vi "Read me and Help.vi"(7 "path":path, 11 "error in":errorcluster) -> (15 "error out":errorcluster)   [LabVIEW 2012]
uses:
  <vilib>/Platform/browser.llb/Open URL in Default Browser (path).vi
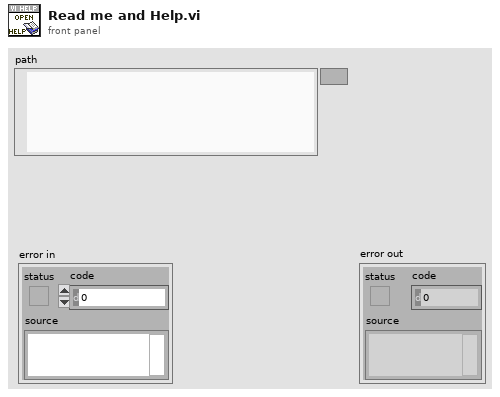
[diagram p1: front panel]
types:
  T1 = enum32{"Invalid", "Standard", "Closed", "Hidden", "Minimized", "Maximized"}
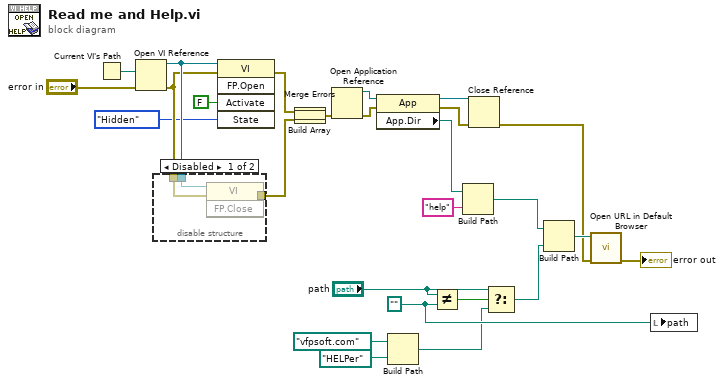
[diagram p0: block diagram]
diagram:
  w12 = path ""
  n1 = Current VI's Path() -> (path=w11:path)
  n2 = Open VI Reference(vi path=w11, error in (no error)="error in") -> (vi reference=w6:refnum<vi>, error out=w5:errorcluster)  [unwired: 4 in]
  n3 = disable-structure shown="Disabled" {
    disable-tunnel: w6 -> [w30 _]
    disable-tunnel: w5 -> [w29 w31]
    disable-tunnel: [w28 w31] -> w10
    frame Disabled {
      n4 = invoke class="VI" method="FP.Close"(reference=w30, error in=w29) -> (error out=w28:errorcluster)  [unwired: 1 in, 2 out]
    }
    frame Enabled {
    }
  }
  n5 = invoke class="VI" method="FP.Open"(reference=w6, error in=w5, "Activate"=FALSE ("Activate?"), "State"=T1."Hidden") -> (error out=w4:errorcluster)  [unwired: 1 in, 4 out]
  n6 = Build Array(w4, w10) -> (w7:errorcluster[])
  n7 = Merge Errors(w7) -> (w8:errorcluster)
  n8 = Open Application Reference(8:w8) -> (0:w21:errorcluster, 3:w20:refnum<vi>)  [unwired: 3 in]
  n9 = property class="App"(reference=w20, error in=w21) -> (reference out=w22:refnum<vi>, error out=w23:errorcluster, "App.Dir"=w24:path)
  n10 = Build Path(base path=path "vfpsoft.com" ("f"), name or relative path=path "HELPer" ("f")) -> (appended path=w1:path)
  n11 = Not Equal?(x="path", y=w12) -> (x != y?=w17:bool)
  n12 = Build Path(base path=w24, name or relative path="help") -> (appended path=w19:path)
  n13 = Close Reference(reference=w22, error in (no error)=w23) -> (error out=w18:errorcluster)
  n14 = Select(t="path", s=w17, f=w1) -> (s? t:f=w15:path)
  n15 = Build Path(base path=w19, name or relative path=w15) -> (appended path=w26:path)
  n16 = call-poly <vilib>:"Open URL in Default Browser.vi"("error in (no error)"=w18, "path"=w26) -> ("error out"=→"error out":errorcluster)  [unwired: 4 in, 1 out]
  n17 = local write "path"(w12) -> ()
